vi "DataCluster_SensorConsole.vi"(8 "error in (no error)":errorcluster) -> (0 "error out":errorcluster, 3 "Data Cluster":T1)   [LabVIEW 2013, in "SensorConsoleLib.lvlib"]
uses:
  SensorConsoleLib.lvlib
  PrivateControls/DataCluster_SensorConsole.ctl
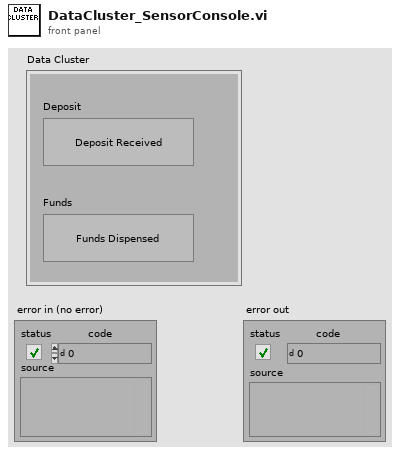
[diagram p1: front panel]
types:
  T1 = typedef "SensorConsoleLib.lvlib/DataCluster_SensorConsole.ctl" = cluster{"Deposit":bool, "Funds":bool}
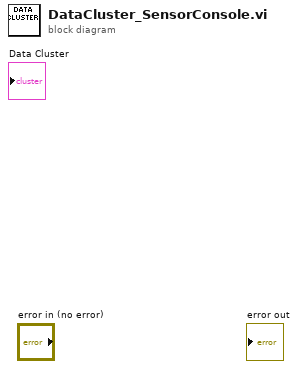
[diagram p0: block diagram]
diagram:
